vi "transition_comparison.vi"(4 "previous_state":T1, 6 "current_state":T1, 7 "transition_queue":refnum<queue>, 8 "error in (no error)":errorcluster, 9 "step":string, 10 "index in":i32, 11 "recipe_data in":variant) -> (0 "error out":errorcluster, 2 "index out":i32, 3 "recipe_data out":variant)   [LabVIEW 2015, in "lv-recipe-machine.lvlib" / "example_01.lvlib"]
doc: "transition_comparison.vi will provide transition functionality for the comparison recipe."
uses:
  example_01.lvlib
  public/_controls/automatic_state.ctl
  public/_controls/transition.ctl
  lv-recipe-machine.lvlib
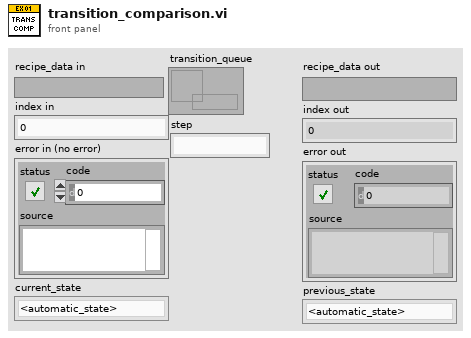
[diagram p1: front panel]
types:
  T1 = typedef "lv-recipe-machine.lvlib/automatic_state.ctl" = enum16{"<automatic_state>", "failed", "idle", "running", "paused", "stopped", "<null>"}
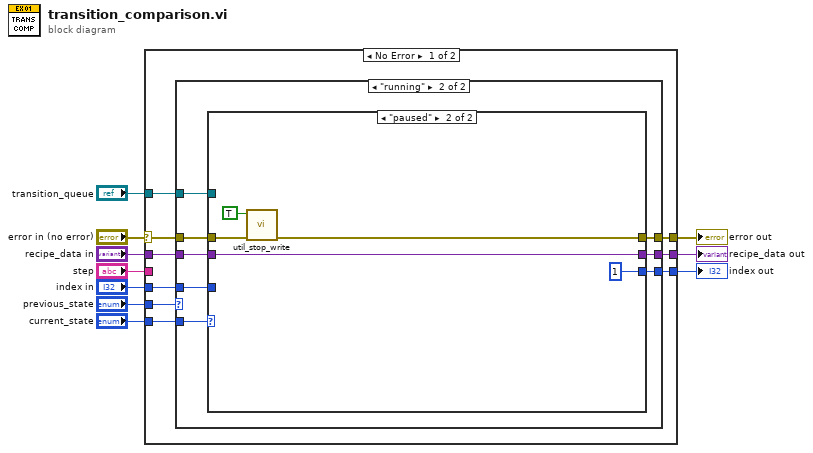
[diagram p0: block diagram]
diagram:
  n1 = case shown="No Error" "error in (no error)" {
    selector: "error in (no error)" -> [w17 w49]
    tunnel: [w16 w49] -> w9
    tunnel: "recipe_data in" -> [w15 w48]
    tunnel: "index in" -> [w13 w47]
    tunnel: "current_state" -> [w18 _]
    tunnel: "previous_state" -> [w19 _]
    tunnel: [w14 w48] -> w4
    tunnel: [w12 w47] -> w3
    tunnel: "transition_queue" -> [w11 _]
    tunnel: "step" -> [_ _]
    frame No Error {
      n2 = case shown="\"running\"" w19 {
        tunnel: w18 -> [w27 w38]
        tunnel: w17 -> [w23 w34]
        tunnel: [w22 w33] -> w16
        tunnel: w15 -> [w25 w36]
        tunnel: [w24 w35] -> w14
        tunnel: w13 -> [w21 w32]
        tunnel: [w20 w31] -> w12
        tunnel: w11 -> [w26 w37]
        frame Default {
          n3 = case shown="Default" w27 {
            tunnel: w26 -> [_]
            tunnel: w25 -> [w30]
            tunnel: [w30] -> w24
            tunnel: w23 -> [w29]
            tunnel: [w29] -> w22
            tunnel: w21 -> [w28]
            tunnel: [w28] -> w20
            frame Default {
            }
          }
        }
        frame "running" {
          n4 = case shown="\"paused\"" w38 {
            tunnel: w37 -> [_ _]
            tunnel: w36 -> [w41 w46]
            tunnel: [w41 w46] -> w35
            tunnel: w34 -> [w40 w44]
            tunnel: [w40 w42] -> w33
            tunnel: w32 -> [w39 _]
            tunnel: [w39 1 ("index in")] -> w31
            frame Default {
            }
            frame "paused" {
              n5 = call "util_stop_write.vi"("error in (no error)"=w44, "stop"=TRUE) -> ("error out"=w42:errorcluster)  [unwired: 9 in]
            }
          }
        }
      }
    }
    frame Error {
    }
  }
  "error out" <- w9
  "recipe_data out" <- w4
  "index out" <- w3
